vi "RTS.vi"(1 "Reg. Select":u8, 2 "SPI Config In":T1) -> (0 "SPI Config Out":T1)   [LabVIEW 2019]
uses:
  SPI/SPI Config.ctl
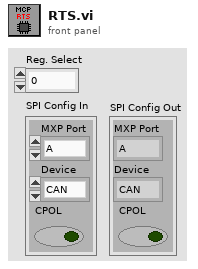
[diagram p1: front panel]
types:
  T1 = typedef "SPI Config.ctl" = cluster{"MXP Port":enum16{"A", "B"}, "Device":enum16{"CAN", "ENC", "IMU1", "IMU2"}, "CPOL":bool}
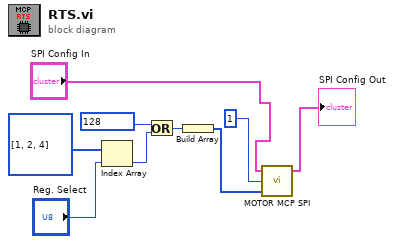
[diagram p0: block diagram]
diagram:
  n1 = Index Array(array=u8[] [1, 2, 4], index="Reg. Select") -> (element=w7:u8)
  n2 = Or(x=u8 128, y=w7) -> (x .or. y?=w9:u8)
  n3 = Build Array(w9) -> (w1:u8[])
  n4 = call "MOTOR MCP SPI.vi"("Data to Write"=w1, "Frames to Write"=u8 1, "SPI Config In"="SPI Config In") -> ("SPI Config Out"=→"SPI Config Out":T1)  [unwired: 2 out]
